vi "RFH-read-R140.vi"(7 "file path (dialog if empty)":path, 8 "error in (no error)":errorcluster) -> (0 "error out":errorcluster, 1 "R140 data":T2, 2 "Common Format":T1)   [LabVIEW 2020, in "RFH-Reflection_File_Handler.lvlib"]
uses:
  RFH-Reflection_File_Handler.lvlib
  RFH-R140_data_format.ctl
  RFH-common_data_format.ctl
  <vilib>/addons/_office/excel.llb/Excel Get Data ([dbl]).vi
  <vilib>/Utility/NIReport.llb/NI_report.lvclass
  <vilib>/Utility/NIReport.llb/Excel/NI_Excel.lvclass
  <vilib>/addons/_office/NI_ReportGenerationToolkit.lvlib
panel:
  out "Frequency":dbl[](graph)
  out "Sheet 1 Data":dbl[][](array[numeric]) format="%.2f"
  out "Output":dbl[][](array[numeric])
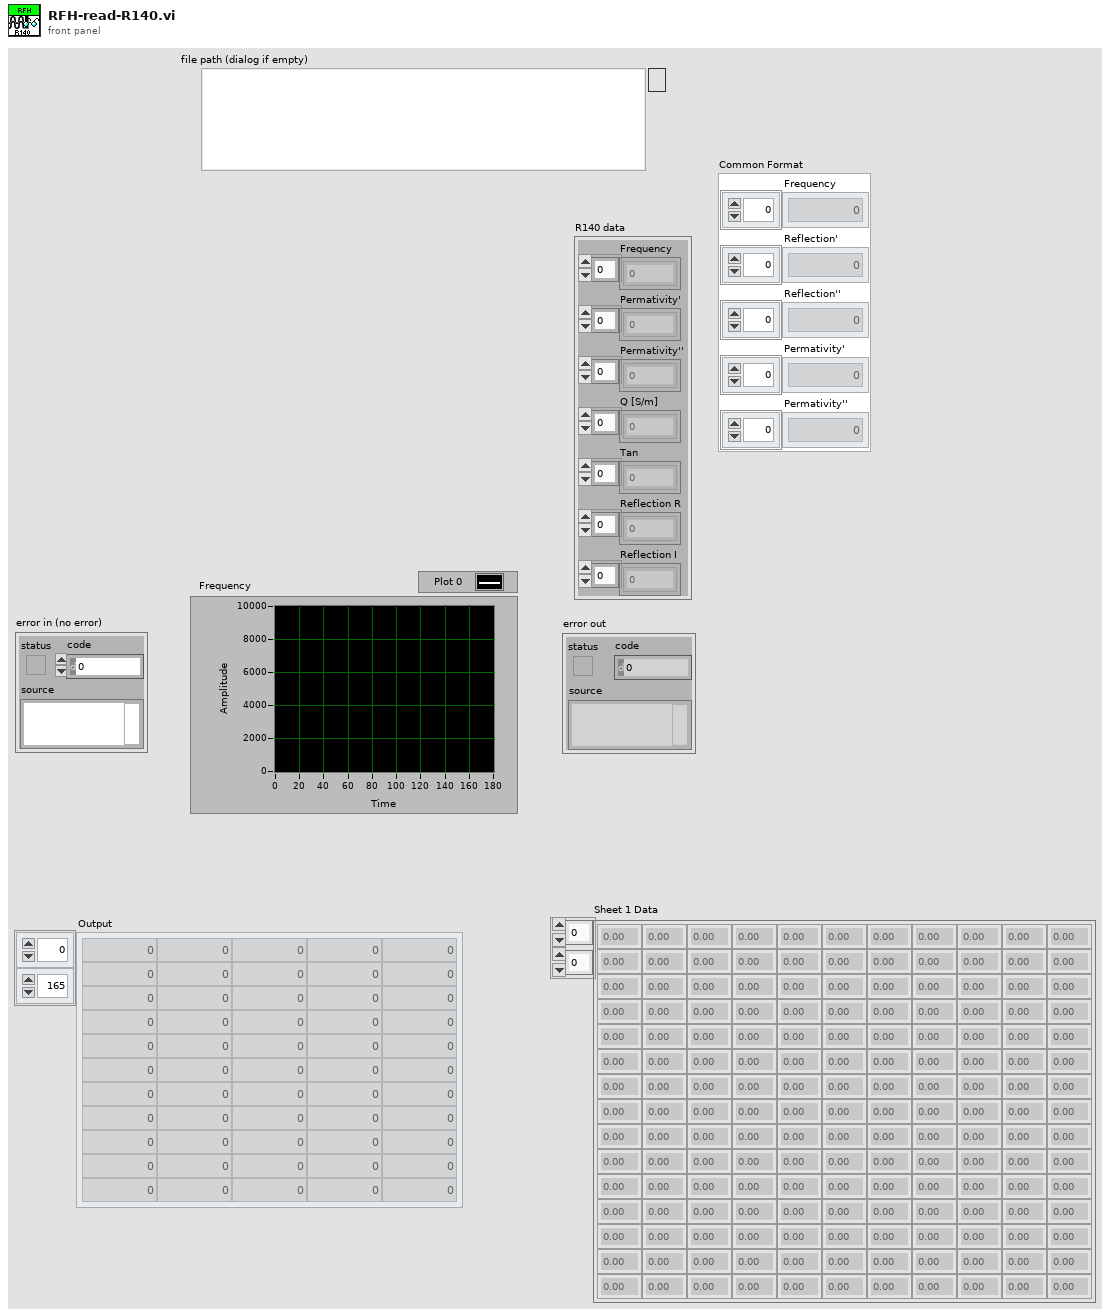
[diagram p1: front panel]
types:
  T1 = typedef "RFH-Reflection_File_Handler.lvlib/RFH-common_data_format.ctl" = cluster{"Frequency":dbl[], "Reflection'":dbl[], "Reflection''":dbl[], "Permativity'":dbl[], "Permativity''":dbl[]}
  T2 = typedef "RFH-Reflection_File_Handler.lvlib/RFH-R140_data_format.ctl" = cluster{"Frequency":dbl[], "Permativity'":dbl[], "Permativity''":dbl[], "Q [S/m]":dbl[], "Tan":dbl[], "Reflection R":dbl[], "Reflection I":dbl[]}
  T3 = enum16{"Standard Report", "HTML", "Word", "Excel"}
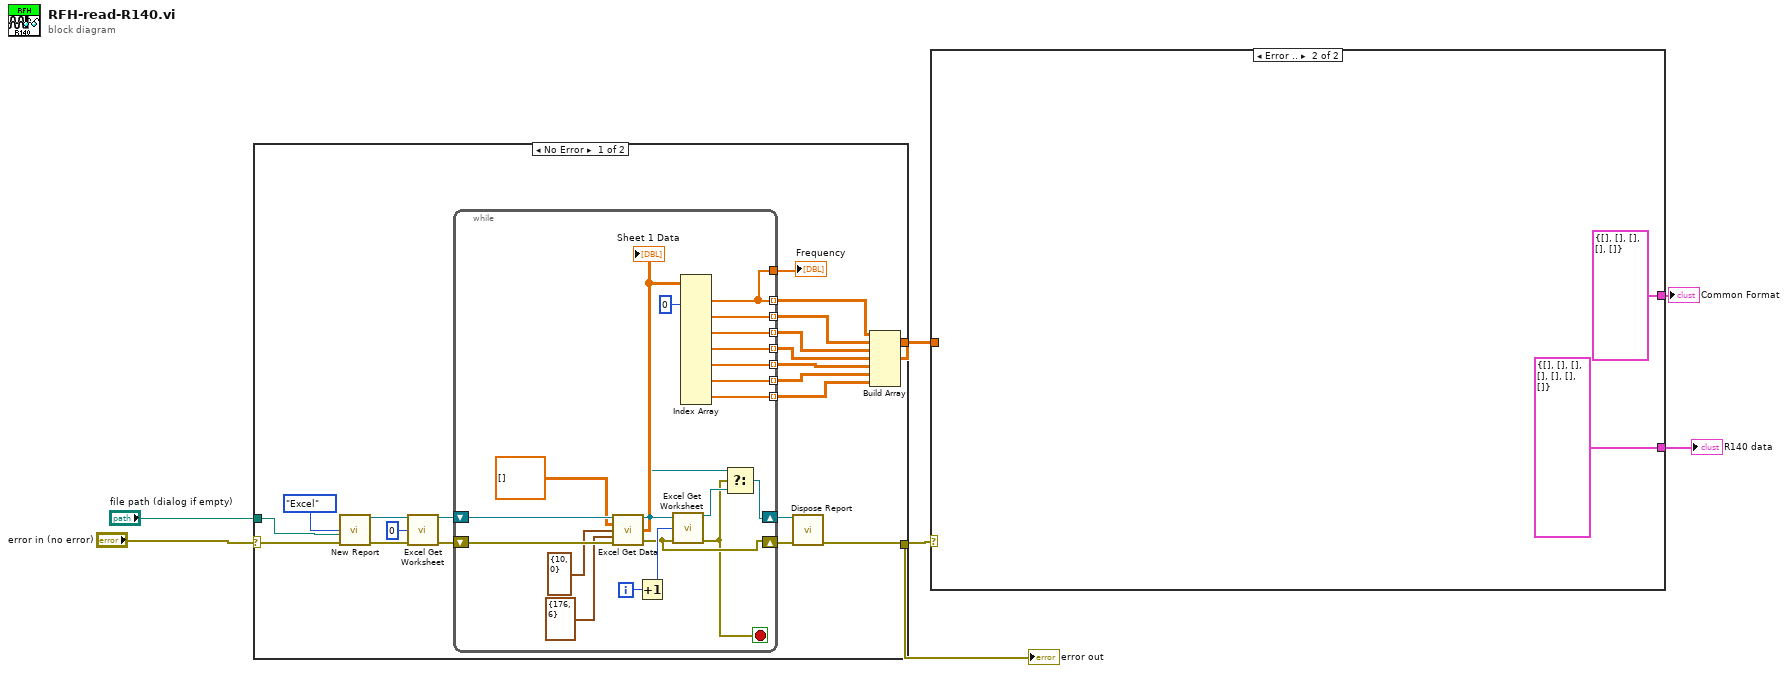
[diagram p0: block diagram]
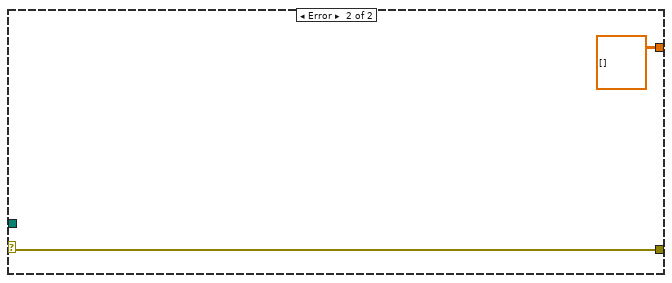
[diagram p2: hidden frame]
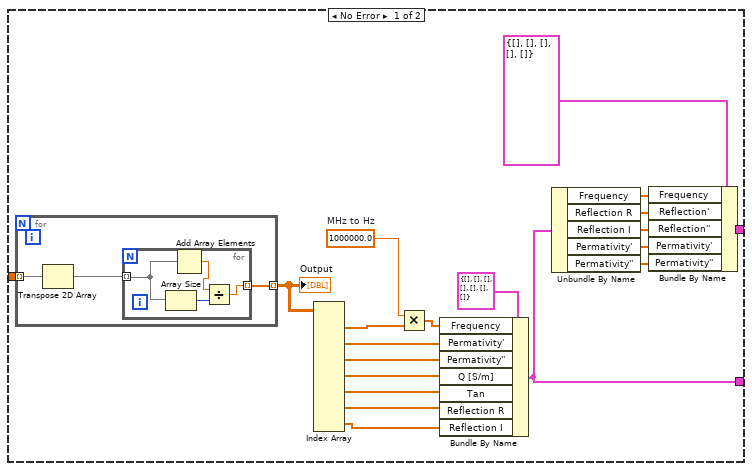
[diagram p3: hidden frame]
diagram:
  n1 = case shown="No Error" "error in (no error)" {
    selector: "error in (no error)" -> [w14 w49]
    tunnel: "file path (dialog if empty)" -> [w23 _]
    tunnel: [w20 dbl[][][] []] -> w5
    tunnel: [w7 w49] -> w1
    frame No Error {
      n2 = call <vilib>:"New Report.vi"("report type"=T3."Excel", "template (empty)"=w23, "error in (no error)"=w14) -> ("report out"=w13:refnum<class "NI_report.lvclass">, "error out"=w12:errorcluster)  [unwired: 3 in, 8 out]
      n3 = call <vilib>:"Excel Get Worksheet.vi"("report in"=w13, "worksheet index (0)"=0, "error in (no error)"=w12) -> ("report out"=w10:refnum<class "NI_report.lvclass">, "error out"=w9:errorcluster)  [unwired: 11 out]
      n4 = while {
        shift-right: [w29] -> w25
        shift-left: w10 -> [w47]
        shift-right: [w32] -> w24
        shift-left: w9 -> [w45]
        tunnel: [w27] -> w22 mode=indexing
        tunnel: [w40] -> w21 mode=indexing
        tunnel: [w39] -> w19 mode=indexing
        tunnel: [w38] -> w18 mode=indexing
        tunnel: [w37] -> w17 mode=indexing
        tunnel: [w36] -> w16 mode=indexing
        tunnel: [w35] -> w15 mode=indexing
        tunnel: [w27] -> w8
        i -> [w34]
        stop <- w28 stop-if-true
        n5 = call-poly <vilib>:"Excel Get Data.vi"("report in"=w47, "data type"=dbl[][] [], "start (-1, -1)"=cluster{"row":i32, "column":i32} {"row"=10, "column"=0}, "end (-1, -1)"=cluster{"row":i32, "column":i32} {"row"=176, "column"=6}, "error in (no error)"=w45) -> ("report out"=w31:refnum<class "NI_report.lvclass">, "data"=w41:dbl[][], "error out"=w32:errorcluster)  [unwired: 8 out]
        "Sheet 1 Data" <- w41
        n6 = Increment(x=w34) -> (x+1=w33:i32)
        n7 = call <vilib>:"Excel Get Worksheet.vi"("report in"=w31, "worksheet index (0)"=w33, "error in (no error)"=w32) -> ("report out"=w30:refnum<class "NI_report.lvclass">, "error out"=w28:errorcluster)  [unwired: 11 out]
        n8 = Index Array(array=w41, index (col) #1=0 ("disabled index (col)")) -> (element #1=w27:dbl[], element #2=w40:dbl[], element #3=w39:dbl[], element #4=w38:dbl[], element #5=w37:dbl[], element #6=w36:dbl[], element #7=w35:dbl[])  [unwired: 13 in]
        n9 = Select(t=w31, s=w28, f=w30) -> (s? t:f=w29:refnum<class "NI_report.lvclass">)
      }
      "Frequency" <- w8
      n10 = call-dynamic "Dispose Report.vi"("report in"=w25, "error in (no error)"=w24) -> ("error out"=w7:errorcluster)  [unwired: 3 in, 10 out]
      n11 = Build Array(w22, w21, w19, w18, w17, w16, w15) -> (w20:dbl[][][])
    }
    frame Error {
    }
  }
  "error out" <- w1
  n12 = case shown="Error .." w1 {
    tunnel: w5 -> [w69 _]
    tunnel: [w57 T2 {"Frequency"=[], "Permativity'"=[], "Permativity''"=[], "Q [S/m]"=[], "Tan"=[], "Reflection R"=[], "Reflection I"=[]} ("output cluster")] -> w3
    tunnel: [w50 T1 {"Frequency"=[], "Reflection'"=[], "Reflection''"=[], "Permativity'"=[], "Permativity''"=[]} ("Common Format")] -> w2
    frame No Error {
      w58 = 1000000.0  # MHz to Hz
      n13 = for {
        tunnel: w69 -> [w70] mode=indexing
        tunnel: [w71] -> w68 mode=indexing
        n14 = Transpose 2D Array(2D array=w70) -> (transposed array=w72:dbl[][])
        n15 = for {
          tunnel: w72 -> [w76] mode=indexing
          tunnel: [w75] -> w71 mode=indexing
          n16 = Array Size(array=w76) -> (size(s)=w73:i32)
          n17 = Add Array Elements(numeric array=w76) -> (sum=w74:dbl)
          n18 = Divide(x=w74, y=w73) -> (x/y=w75:dbl)
        }
      }
      "Output" <- w68
      n19 = Index Array(array=w68) -> (element #1=w67:dbl[], element #2=w66:dbl[], element #3=w65:dbl[], element #4=w64:dbl[], element #5=w63:dbl[], element #6=w62:dbl[], element #7=w61:dbl[])  [unwired: 14 in]
      n20 = Multiply(x=w58, y=w67) -> (x*y=w59:dbl[])
      n21 = Bundle By Name(cluster=T2 {"Frequency"=[], "Permativity'"=[], "Permativity''"=[], "Q [S/m]"=[], "Tan"=[], "Reflection R"=[], "Reflection I"=[]} ("output cluster"), "Frequency"=w59, "Permativity'"=w66, "Permativity''"=w65, "Q [S/m]"=w64, "Tan"=w63, "Reflection R"=w62, "Reflection I"=w61) -> (w57:T2)
      n22 = Unbundle By Name(w57) -> ("Frequency"=w55:dbl[], "Reflection R"=w54:dbl[], "Reflection I"=w53:dbl[], "Permativity'"=w52:dbl[], "Permativity''"=w51:dbl[])
      n23 = Bundle By Name(cluster=T1 {"Frequency"=[], "Reflection'"=[], "Reflection''"=[], "Permativity'"=[], "Permativity''"=[]} ("Common Format"), "Frequency"=w55, "Reflection'"=w54, "Reflection''"=w53, "Permativity'"=w52, "Permativity''"=w51) -> (w50:T1)
    }
    frame Error {
    }
  }
  "R140 data" <- w3
  "Common Format" <- w2
